vi "MC.TestLauncher.vi"() -> ()   [LabVIEW 2017, in "MC.lvclass"]
doc: "JKI State Machine Objects (SMO) 1.0.0.5\nJKI - JKI\nCopyright (c) 2016, JKI"
uses:
  MC.lvclass
  <vilib>/JKI/JKI SMO/SMO/Typedefs/SMOState --Enum.ctl
  D:/Program Files (x86)/National Instruments/LabVIEW 2017/vi.lib/JKI/JKI SMO/SMO/SMO.lvclass
  <vilib>/JKI/JKI SMO/SMO/SMO.lvclass
panel:
  out "State":T1
  out "error out":errorcluster
  in  "Stop":bool
  # "Basic SMO byRef Test Launcher"
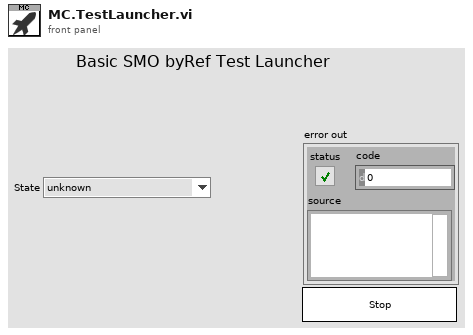
[diagram p1: front panel]
types:
  T1 = typedef "SMO.lvclass/SMOState --Enum.ctl" = enum16{"unknown", "Created", "Started", "Stopped"}
  T2 = typedef "SMO.lvclass/Public Events.ctl" = cluster{"Error":refnum<user-event>, "State":refnum<user-event>, "Reserve State":refnum<user-event>}
  T3 = cluster{"Event Registration Refnum":refnum<event-registration>}
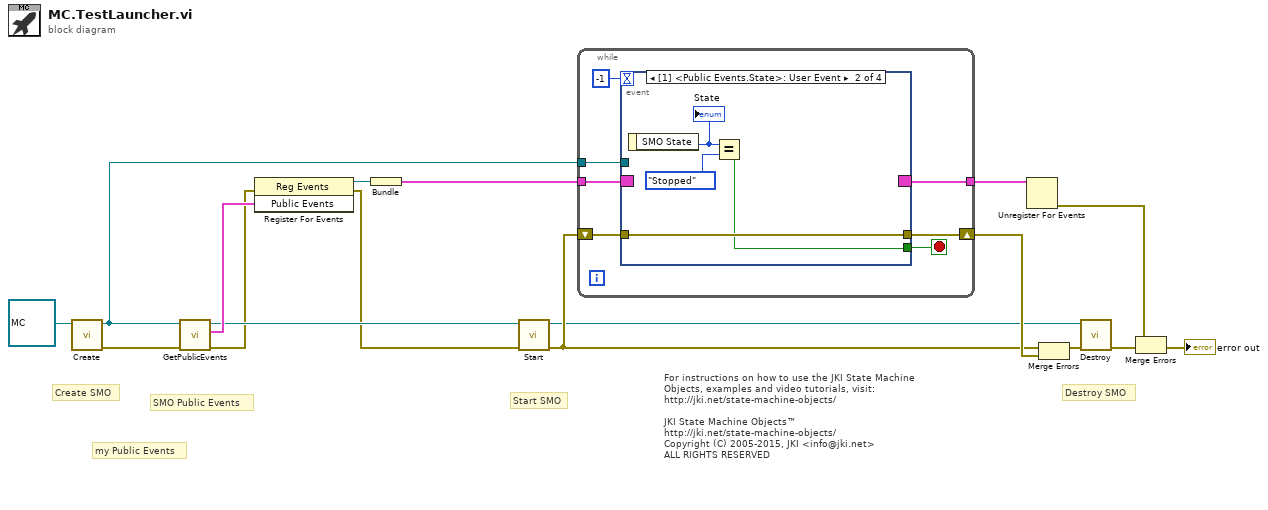
[diagram p0: block diagram]
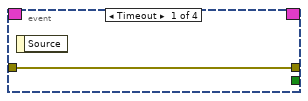
[diagram p2: hidden frame]
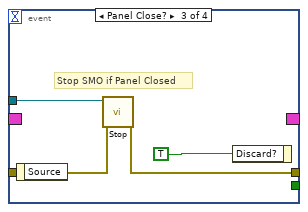
[diagram p3: hidden frame]
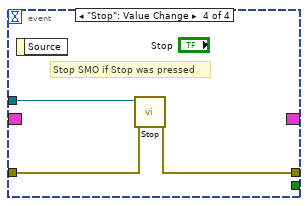
[diagram p4: hidden frame]
diagram:
  # "SMO Public Events"
  # "For instructions on how to use the JKI State Machine Objects, examples and video tutorials, visit:\nhttp://jki.net/state-machine-objects/\n\nJKI State Machine Objects™\nhttp://jki.net/state-machine-objects/\nCopyright (C) 2005-2015, JKI <info@jki.net>\nALL RIGHTS RESERVED"
  # "my Public Events"
  # "Start SMO"
  # "Destroy SMO"
  # "Create SMO"
  n1 = call <vilib>:"Create.vi"("SMO"=refnum<class "MC.lvclass"> refnum ("SMO.Template.lvclass")) -> ("error out"=w1:errorcluster, "SMO out"=w8:refnum<class "MC.lvclass">)  [unwired: 8 in, 1 out]
  n2 = call <vilib>:"GetPublicEvents.vi"("error in (no error)"=w1, "SMO"=w8) -> ("error out"=w5:errorcluster, "Public Events"=w7:T2, "SMO out"=w6:refnum<class "MC.lvclass">)  [unwired: 7 in]
  n3 = register-events(error in=w5, w7) -> (reference out=w9:refnum<event-registration>, error out=w4:errorcluster)  [unwired: 1 in]
  n4 = Bundle("Event Registration Refnum"=w9) -> (w16:T3)  [unwired: 1 in]
  n5 = call <vilib>:"Start.vi"("error in (no error)"=w4, "SMO"=w6) -> ("error out"=w10:errorcluster, "SMO out"=w2:refnum<class "MC.lvclass">)  [unwired: 8 in]
  n6 = while {
    shift-right: [w23] -> w15
    shift-left: w10 -> [w22]
    tunnel: w16 -> [w21]
    tunnel: [w20] -> w17
    tunnel: w8 -> [w19]
    stop <- w24 stop-if-true
    n7 = event shown="[1] <Public Events.State>: User Event" {
      selector: w21 -> [_ _ _ _]
      dyn-events: [_ _ _ _] -> w20
      timeout: -1 -> [_ _ _ _]
      tunnel: [_ w26 _ _] -> w24
      tunnel: w19 -> [_ _ w33 w36]
      tunnel: [w25 w29 w32 w35] -> w23
      tunnel: w22 -> [w25 w29 w31 w34]
      event Timeout {
        n8 = event-data() -> ()  [unwired: 1 in, 1 out]
      }
      event User Event {
        n9 = event-data() -> ("SMO State"=w28:T1)  [unwired: 1 in]
        "State" <- w28
        n10 = Equal?(x=w28, y=SMOState_--Enum."Stopped") -> (x = y?=w26:bool)
      }
      event Panel Close? {
        # "Stop SMO if Panel Closed"
        n11 = event-data() -> ()  [unwired: 1 in, 1 out]
        n12 = call <vilib>:"Stop.vi"("error in (no error)"=w31, "SMO"=w33) -> ("error out"=w32:errorcluster)  [unwired: 8 in, 1 out]
        n13 = event-data("Discard?"=TRUE ("OK")) -> ()  [unwired: 1 in, 1 out]
      }
      event "Stop": Value Change {
        # "Stop SMO if Stop was pressed"
        n14 = event-data() -> ()  [unwired: 1 in, 1 out]
        n15 = call <vilib>:"Stop.vi"("error in (no error)"=w34, "SMO"=w36) -> ("error out"=w35:errorcluster)  [unwired: 8 in, 1 out]
      }
    }
  }
  n16 = Unregister For Events(event registration refnum=w17) -> (error out=w14:errorcluster)  [unwired: 1 in]
  n17 = Merge Errors(w10, w15) -> (w3:errorcluster)
  n18 = call <vilib>:"Destroy.vi"("error in (no error)"=w3, "SMO"=w2) -> ("error out"=w12:errorcluster)  [unwired: 9 in]
  n19 = Merge Errors(w14, w12) -> (→"error out":errorcluster)
